vi "Get Scalar Datatypes and Refs.vi"(8 "error in (no error)":errorcluster, 9 "FPGA Ref":refnum<k20>, 10 "Item GUID":string, 11 "Section Ref in":T4 format="%.0x") -> (0 "error out":errorcluster, 1 "FPGA Ref":refnum<k20>, 2 "VS Ref":T4[](array[typedef]) format="%.0x", 3 "Section Ref out":T4 format="%.0x", 4 "Registers Ref":T1[](array[typedef]) {"Data Type" format="%.0x"})   [LabVIEW 2013, in "FPGA Addon Engine.lvlib"]
uses:
  FPGA Addon Engine.lvlib
  <vilib>/NI Veristand/Custom Device API/Custom Device Item Ref.ctl
  Types/Register Settings.ctl
  <userlib>/_OpenG.lib/lvdata/lvdata.llb/Type Descriptor Enumeration__ogtk.ctl
  Shared/Scalar Type.ctl
  Shared/FG Action.ctl
  <vilib>/NI Veristand/Custom Device Tools/Custom Device Utility Library/NI VeriStand - Search for Item by GUID.vi
  Shared/Constants.vi
  <vilib>/NI Veristand/Custom Device API/Get Item Property (Variant).vi
  <vilib>/NI Veristand/Custom Device API/Get Item Property (String).vi
  Shared/FPGA Addon Shared.lvlib
  <vilib>/NI VeriStand/Custom Device API/Custom Device API.lvlib
  <vilib>/NI Veristand/Custom Device Tools/Custom Device Utility Library/Custom Device Utility Library.lvlib
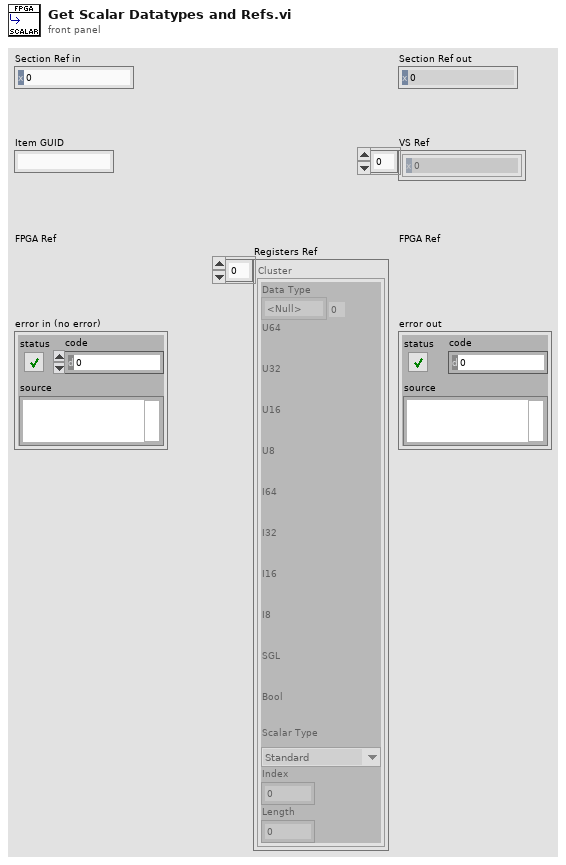
[diagram p1: front panel]
types:
  T1 = typedef "FPGA Addon Engine.lvlib/Register Settings.ctl" = cluster{"Data Type":T2, "U64":refnum<k20>, "U32":refnum<k20>, "U16":refnum<k20>, "U8":refnum<k20>, "I64":refnum<k20>, "I32":refnum<k20>, "I16":refnum<k20>, "I8":refnum<k20>, "SGL":refnum<k20>, "Bool":refnum<k20>, "Scalar Type":T3, "Index":i32, "Length":i32}
  T2 = typedef "Type Descriptor Enumeration__ogtk.ctl" = enum8{"<Null>", "I8", "I16", "I32", "I64", "U8", "U16", "U32", "U64", "SGL", "DBL", "EXT", "CSG", "CDB", "CXT", "0x0F", "0x10", "0x11", "0x12", "0x13", "0x14", "Enum U8", "Enum U16", "Enum U32", "Enum U64", "SGL PQ", "DBL PQ", "EXT PQ", "CSG PQ", "CDB PQ", "CXT PQ", "0x1F", "0x20", "Boolean", "0x22", "0x23", "0x24", "0x25", "0x26", "0x27", "0x28", "0x29", "0x2A", "0x2B", "0x2C", "0x2D", "0x2E", "0x2F", "String", "0x31", "Path", "Pict", "0x34", "0x35", "0x36", "DAQ", "0x38", "0x39", "0x3A", "0x3B", "0x3C", "0x3D", "0x3E", "0x3F", "Array", "0x41", "0x42", "0x43", "0x44", "0x45", "0x46", "0x47", "0x48", "0x49", "0x4A", "0x4B", "0x4C", "0x4D", "0x4E", "0x4F", "Cluster", "0x51", "0x52", "Variant", "Waveform", "0x55", "0x56", "0x57", "0x58", "0x59", "0x5A", "0x5B", "0x5C", "0x5D", "0x5E", "0x5F", "0x60", "0x61", "0x62", "0x63", "0x64", "0x65", "0x66", "0x67", "0x68", "0x69", "0x6A", "0x6B", "0x6C", "0x6D", "0x6E", "0x6F", "Refnum"}
  T3 = typedef "FPGA Addon Shared.lvlib/Scalar Type.ctl" = enum16{"Standard", "Bitpacked"}
  T4 = typedef "Custom Device API.lvlib/Custom Device Item Ref.ctl" = u64
  T5 = typedef "FPGA Addon Shared.lvlib/FG Action.ctl" = enum8{"GET", "SET"}
  T6 = typedef "FPGA Addon Shared.lvlib/Register Information.ctl" = cluster{"Name":string, "Data Type":T2, "Default Value":dbl}
  T7 = typedef "Custom Device API.lvlib/Custom Device Item Info.ctl" = cluster{"Name":string, "Is Channel":bool, "GUID":string, "Is Waveform":bool}
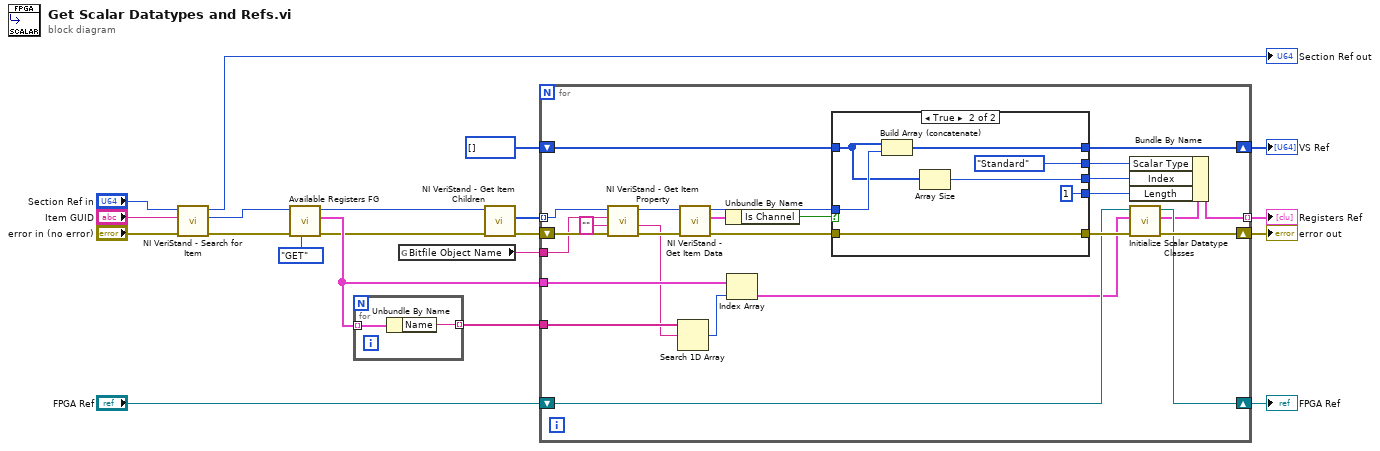
[diagram p0: block diagram]
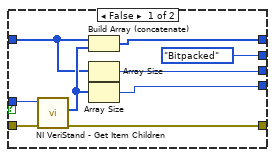
[diagram p2: hidden frame]
diagram:
  n1 = call-poly <vilib>:"NI VeriStand - Search for Item.vi"("error in"="error in (no error)", "Item GUID"="Item GUID", "Section Ref in"="Section Ref in") -> ("error out"=w16:errorcluster, "Item Ref"=w18:T4, "Section Ref out"=→"Section Ref out":T4)  [unwired: 5 in, 1 out]
  n2 = call "Available Registers FG.vi"("Action"=FG_Action."GET", "error in (no error)"=w16, "Item Ref"=w18) -> ("error out"=w12:errorcluster, "Available Registers"=w13:T6[], "Item Ref out"=w14:T4)  [unwired: 6 in]
  n3 = for {
    tunnel: w13 -> [w22] mode=indexing
    tunnel: [w21] -> w11 mode=indexing
    n4 = Unbundle By Name(w22) -> ("Name"=w21:string)
  }
  n5 = global read "Constants.vi" "Bitfile Object Name"() -> (w10:string)
  n6 = call <vilib>:"NI VeriStand - Get Item Children.vi"("error in (no error)"=w12, "Item Ref in"=w14) -> ("error out"=w8:errorcluster, "Child Refs"=w9:T4[])  [unwired: 6 in, 2 out]
  n7 = for {
    shift-right: [w34] -> w4
    shift-left: w8 -> [w48]
    tunnel: w9 -> [w47] mode=indexing
    tunnel: w10 -> [w46]
    tunnel: w11 -> [w44]
    tunnel: w13 -> [w42]
    shift-right: [w32] -> w2
    shift-left: "FPGA Ref" -> [w33]
    shift-right: [w29] -> w5
    shift-left: T4[] [] -> [w30]
    tunnel: [w27] -> w6 mode=indexing
    n8 = call-poly <vilib>:"NI VeriStand - Get Item Property.vi"("error in (no error)"=w48, "Default Value"="", "Property Name"=w46, "Item Ref in"=w47) -> ("error out"=w40:errorcluster, "Value"=w26:string, "Item Ref out"=w43:T4)  [unwired: 4 in, 1 out]
    n9 = Search 1D Array(1D array=w44, element=w26) -> (index of element=w41:i32)  [unwired: 1 in]
    n10 = call <vilib>:"NI VeriStand - Get Item Data.vi"("error in (no error)"=w40, "Item Ref in"=w43) -> ("error out"=w37:errorcluster, "Item Info"=w39:T7, "Item Ref out"=w38:T4)  [unwired: 6 in, 1 out]
    n11 = Unbundle By Name(w39) -> ("Is Channel"=w36:bool)
    n12 = Index Array(array=w42, index=w41) -> (element=w31:T6)
    n13 = case shown="True" w36 {
      tunnel: w38 -> [w56 w63]
      tunnel: w37 -> [w57 w64]
      tunnel: [w55 w64] -> w35
      tunnel: w30 -> [w52 w60]
      tunnel: [w53 w62] -> w29
      tunnel: [Scalar_Type."Bitpacked" ("Scalar Type") Scalar_Type."Standard" ("Scalar Type")] -> w25
      tunnel: [w51 w59] -> w24
      tunnel: [w50 1] -> w23
      frame False {
        n14 = call <vilib>:"NI VeriStand - Get Item Children.vi"("error in (no error)"=w57, "Item Ref in"=w56) -> ("error out"=w55:errorcluster, "Child Refs"=w54:T4[])  [unwired: 6 in, 2 out]
        n15 = Build Array (concatenate)(w52, w54) -> (w53:T4[])
        n16 = Array Size(array=w52) -> (size(s)=w51:i32)
        n17 = Array Size(array=w54) -> (size(s)=w50:i32)
      }
      frame True {
        n18 = Build Array (concatenate)(w60, w63) -> (w62:T4[])
        n19 = Array Size(array=w60) -> (size(s)=w59:i32)
      }
    }
    n20 = call "Initialize Scalar Datatype Classes.vi"("error in (no error)"=w35, "Register"=w31, "FPGA Ref"=w33) -> ("error out"=w34:errorcluster, "Register"=w28:T1, "FPGA Ref"=w32:refnum<k20>)  [unwired: 6 in]
    n21 = Bundle By Name(cluster=w28, "Scalar Type"=w25, "Index"=w24, "Length"=w23) -> (w27:T1)
  }
  "error out" <- w4
  "VS Ref" <- w5
  "Registers Ref" <- w6
  "FPGA Ref" <- w2
